vi "Create Sense Reference Read.vi"(8 "error in (no error)":errorcluster, 11 "Device Item Ref in":T1 format="%.0x") -> (0 "error out":errorcluster)   [LabVIEW 2020, in "G5 Regatron Custom Device System Explorer.lvlib"]
uses:
  G5 Regatron Custom Device System Explorer.lvlib
  <vilib>/NI VeriStand/Custom Device API/Custom Device API.lvlib
  <vilib>/NI VeriStand/Custom Device API/Custom Device Channel Type.ctl
  <vilib>/NI VeriStand/Custom Device API/Custom Device Channel.ctl
  <vilib>/NI VeriStand/Custom Device API/Custom Device Item Ref.ctl
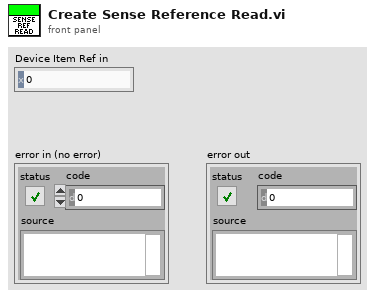
[diagram p1: front panel]
types:
  T1 = typedef "Custom Device API.lvlib/Custom Device Item Ref.ctl" = u64
  T2 = typedef "Custom Device API.lvlib/Custom Device Channel.ctl" = cluster{"Type":T3, "Units":string, "Default Value":dbl, "Faultable":bool, "Scalable":bool}
  T3 = typedef "Custom Device API.lvlib/Custom Device Channel Type.ctl" = enum16{"Input", "Output"}
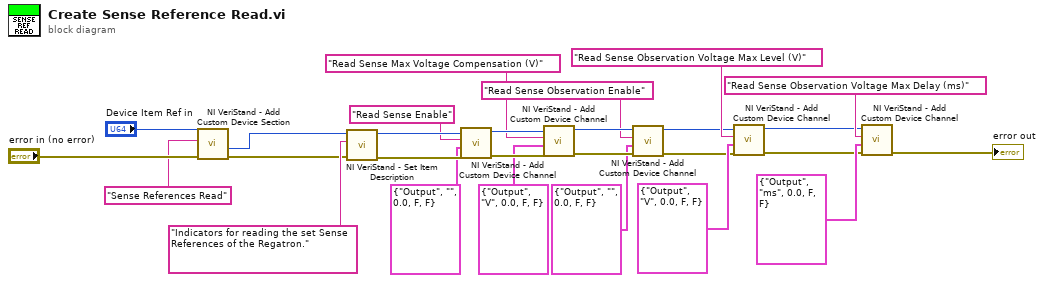
[diagram p0: block diagram]
diagram:
  n1 = call <vilib>:"NI VeriStand - Add Custom Device Section.vi"("error in (no error)"="error in (no error)", "Section Name"="Sense References Read", "Parent Ref in"="Device Item Ref in") -> ("error out"=w23:errorcluster, "Section Ptr"=w25:T1)  [unwired: 5 in, 2 out]
  n2 = call <vilib>:"NI VeriStand - Set Item Description.vi"("error in (no error)"=w23, "Description"="Indicators for reading the set Sense References of the Regatron.", "Item Ref in"=w25) -> ("error out"=w24:errorcluster, "Item Ref out"=w26:T1)  [unwired: 6 in, 1 out]
  n3 = call <vilib>:"NI VeriStand - Add Custom Device Channel.vi"("error in (no error)"=w24, "Channel"=T2 {"Type"=enum."Output", "Units"="", "Default Value"=0.0, "Faultable"=FALSE, "Scalable"=FALSE}, "Channel Name"="Read Sense Enable", "Parent Ref in"=w26) -> ("error out"=w16:errorcluster, "Parent Ref out"=w15:T1)  [unwired: 4 in, 2 out]
  n4 = call <vilib>:"NI VeriStand - Add Custom Device Channel.vi"("error in (no error)"=w16, "Channel"=T2 {"Type"=enum."Output", "Units"="V", "Default Value"=0.0, "Faultable"=FALSE, "Scalable"=FALSE}, "Channel Name"="Read Sense Max Voltage Compensation (V)", "Parent Ref in"=w15) -> ("error out"=w12:errorcluster, "Parent Ref out"=w11:T1)  [unwired: 4 in, 2 out]
  n5 = call <vilib>:"NI VeriStand - Add Custom Device Channel.vi"("error in (no error)"=w12, "Channel"=T2 {"Type"=enum."Output", "Units"="", "Default Value"=0.0, "Faultable"=FALSE, "Scalable"=FALSE}, "Channel Name"="Read Sense Observation Enable", "Parent Ref in"=w11) -> ("error out"=w3:errorcluster, "Parent Ref out"=w4:T1)  [unwired: 4 in, 2 out]
  n6 = call <vilib>:"NI VeriStand - Add Custom Device Channel.vi"("error in (no error)"=w3, "Channel"=T2 {"Type"=enum."Output", "Units"="V", "Default Value"=0.0, "Faultable"=FALSE, "Scalable"=FALSE}, "Channel Name"="Read Sense Observation Voltage Max Level (V)", "Parent Ref in"=w4) -> ("error out"=w1:errorcluster, "Parent Ref out"=w2:T1)  [unwired: 4 in, 2 out]
  n7 = call <vilib>:"NI VeriStand - Add Custom Device Channel.vi"("error in (no error)"=w1, "Channel"=T2 {"Type"=enum."Output", "Units"="ms", "Default Value"=0.0, "Faultable"=FALSE, "Scalable"=FALSE}, "Channel Name"="Read Sense Observation Voltage Max Delay (ms)", "Parent Ref in"=w2) -> ("error out"=→"error out":errorcluster)  [unwired: 4 in, 3 out]
